vi "Sending HardWare PreDef Parameters.vi"(8 "VISA resource name":refnum<visa-resource-name>) -> (0 "HArdware OK?":bool)   [LabVIEW 2011]
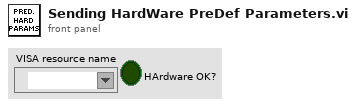
[diagram p1: front panel]
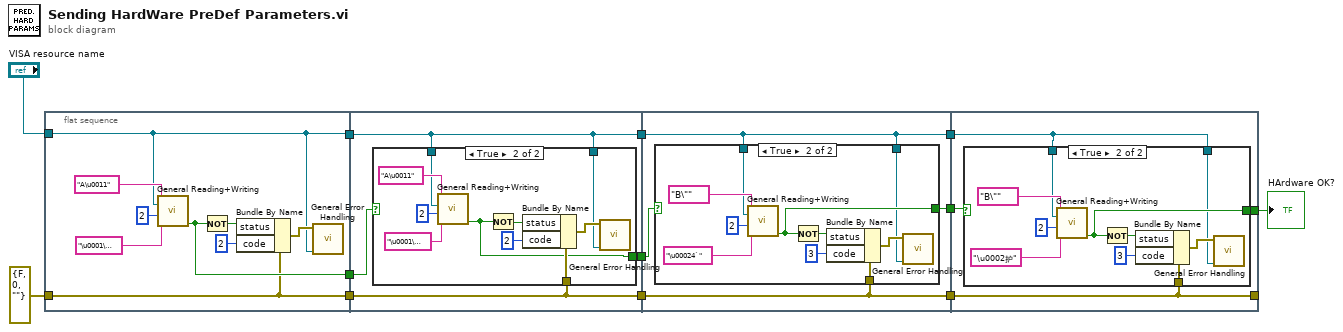
[diagram p0: block diagram]
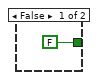
[diagram p2: hidden frame]
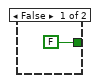
[diagram p3: hidden frame]
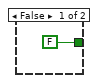
[diagram p4: hidden frame]
diagram:
  n1 = flat-sequence {
    tunnel: "VISA resource name" -> [w13]
    tunnel: [w13] -> w11
    tunnel: [w17] -> w10
    tunnel: errorcluster {"status"=FALSE, "code"=0, "source"=""} ("error IO") -> [w15]
    tunnel: [w15] -> w8
    tunnel: w11 -> [w22]
    tunnel: w10 -> [w25]
    tunnel: w8 -> [w24]
    tunnel: [w22] -> w7
    tunnel: [w24] -> w6
    tunnel: [w23] -> w3
    tunnel: w7 -> [w37]
    tunnel: w6 -> [w39]
    tunnel: [w37] -> w5
    tunnel: [w39] -> w4
    tunnel: w3 -> [w40]
    tunnel: [w38] -> w2
    tunnel: [w54] -> _
    tunnel: w5 -> [w52]
    tunnel: w4 -> [w54]
    tunnel: w2 -> [w55]
    tunnel: [w53] -> w1
    frame #0 {
      n2 = call "General Reading+Writing.vi"("Write String"="\u0001\u0001\u0002" ("write buffer"), "Number Of Bytes to Read"=u32 2, "VISA resource name"=w13, "String Seached"="A\u0011") -> ("Coincidence Of Character"=w17:bool)  [unwired: 4 in, 3 out]
      n3 = Not(x=w17) -> (.not. x?=w16:bool)
      n4 = Bundle By Name(cluster=w15, "status"=w16, "code"=2) -> (w18:errorcluster)
      n5 = call "General Error Handling.vi"("VISA resource name"=w13, "error IO"=w18) -> ()  [unwired: 10 in]
    }
    frame #1 {
      n6 = case shown="True" w25 {
        tunnel: w22 -> [_ w33]
        tunnel: w24 -> [_ w31]
        tunnel: [FALSE ("Coincidence Of Character") w29] -> w23
        tunnel: w22 -> [_ w27]
        frame False {
        }
        frame True {
          n7 = call "General Reading+Writing.vi"("Write String"="\u0001\u0002 " ("write buffer"), "Number Of Bytes to Read"=u32 2, "VISA resource name"=w33, "String Seached"="A\u0011") -> ("Coincidence Of Character"=w29:bool)  [unwired: 4 in, 3 out]
          n8 = Not(x=w29) -> (.not. x?=w30:bool)
          n9 = Bundle By Name(cluster=w31, "status"=w30, "code"=2) -> (w32:errorcluster)
          n10 = call "General Error Handling.vi"("VISA resource name"=w27, "error IO"=w32) -> ()  [unwired: 10 in]
        }
      }
    }
    frame #2 {
      n11 = case shown="True" w40 {
        tunnel: w37 -> [_ w47]
        tunnel: w39 -> [_ w45]
        tunnel: [FALSE ("Coincidence Of Character") w44] -> w38
        tunnel: w37 -> [_ w42]
        frame False {
        }
        frame True {
          n12 = call "General Reading+Writing.vi"("Write String"="\u00024`" ("write buffer"), "Number Of Bytes to Read"=u32 2, "VISA resource name"=w47, "String Seached"="B\"") -> ("Coincidence Of Character"=w44:bool)  [unwired: 4 in, 3 out]
          n13 = Not(x=w44) -> (.not. x?=w43:bool)
          n14 = Bundle By Name(cluster=w45, "status"=w43, "code"=3) -> (w48:errorcluster)
          n15 = call "General Error Handling.vi"("VISA resource name"=w42, "error IO"=w48) -> ()  [unwired: 10 in]
        }
      }
    }
    frame #3 {
      n16 = case shown="True" w55 {
        tunnel: w52 -> [_ w63]
        tunnel: w54 -> [_ w61]
        tunnel: [FALSE ("Coincidence Of Character") w60] -> w53
        tunnel: w52 -> [_ w57]
        frame False {
        }
        frame True {
          n17 = call "General Reading+Writing.vi"("Write String"="\u0002护" ("write buffer"), "Number Of Bytes to Read"=u32 2, "VISA resource name"=w63, "String Seached"="B\"") -> ("Coincidence Of Character"=w60:bool)  [unwired: 4 in, 3 out]
          n18 = Not(x=w60) -> (.not. x?=w59:bool)
          n19 = Bundle By Name(cluster=w61, "status"=w59, "code"=3) -> (w58:errorcluster)
          n20 = call "General Error Handling.vi"("VISA resource name"=w57, "error IO"=w58) -> ()  [unwired: 10 in]
        }
      }
    }
  }
  "HArdware OK?" <- w1
